vi "runFile.vi"() -> ()   [LabVIEW 2017]
panel:
  out "y 2":i32
  out "y":i32
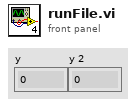
[diagram p1: front panel]
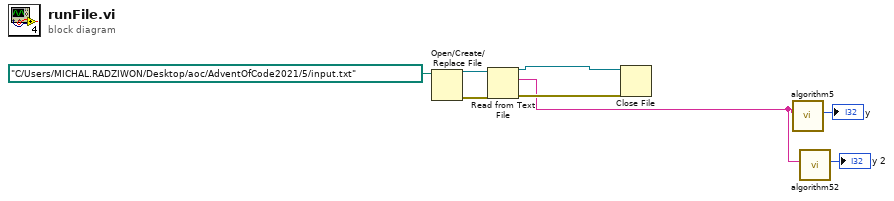
[diagram p0: block diagram]
diagram:
  n1 = Open/Create/Replace File(file path (use dialog)=path "C:/Users/MICHAL.RADZIWON/Desktop/aoc/AdventOfCode2021/5/input.txt") -> (refnum out=w6:refnum<file>, error out=w7:errorcluster)  [unwired: 5 in, 1 out]
  n2 = Read from Text File(file (use dialog)=w6, error in=w7) -> (refnum out=w5:refnum<file>, text=w2:string, error out=w4:errorcluster)  [unwired: 2 in, 1 out]
  n3 = Close File(refnum=w5, error in=w4) -> ()  [unwired: 2 out]
  n4 = call "algorithm5.vi"("String"=w2) -> ("y"=→"y":i32)  [unwired: 10 in]
  n5 = call "algorithm52.vi"("String"=w2) -> ("y"=→"y 2":i32)  [unwired: 10 in]
